vi "Read SpO2.vi"(8 "error in (no error)":errorcluster, 11 "SpO2 Calibration [SpO2/V]":dbl) -> (0 "error out":errorcluster, 2 "Color Out":u32, 3 "SpO2 [%]":dbl)   [LabVIEW 2016]
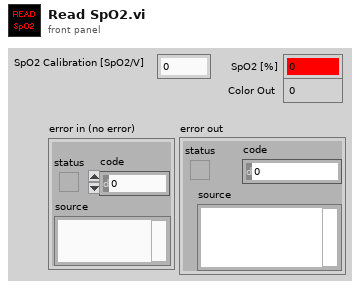
[diagram p1: front panel]
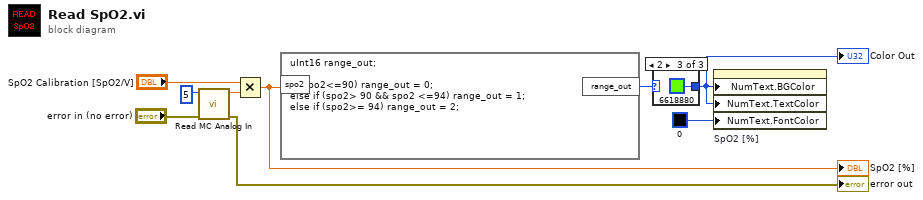
[diagram p0: block diagram]
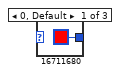
[diagram p2: hidden frame]
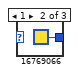
[diagram p3: hidden frame]
diagram:
  n1 = call "Read MC Analog In.vi"("error in (no error)"="error in (no error)", "channel"=5) -> ("error out"=→"error out":errorcluster, "Voltage Input"=w4:dbl)  [unwired: 8 in]
  n2 = Multiply(x="SpO2 Calibration [SpO2/V]", y=w4) -> (x*y=w2:dbl)
  "SpO2 [%]" <- w2
  n3 = formula code="uInt16 range_out;\n\nif (spo2<=90) range_out = 0;\nelse if (spo2> 90 && spo2 <=94) range_out = 1;\nelse if (spo2>= 94) range_out = 2;"("spo2"=w2) -> ("range_out"=w9:u16)
  n4 = case shown="2" w9 {
    tunnel: [u32 16711680 u32 16769066 u32 6618880] -> w7
    frame 0, Default {
    }
    frame 1 {
    }
    frame 2 {
    }
  }
  "Color Out" <- w7
  n5 = property on="SpO2 [%]" class="DigNum (strict)"("NumText.BGColor"=w7, "NumText.TextColor"=w7, "NumText.FontColor"=u32 0) -> ()  [unwired: 2 in, 2 out]
